vi "Exercise 3-6.vi"() -> ()   [LabVIEW 2014]
panel:
  out "Temperature in Desired Measurement":dbl
  in  "Temperature":dbl
  in  "Desired Measurement":enum16{"K", "F", "C"}(ring)
  in  "Temperature Measurment":enum16{"F", "C"}(ring)
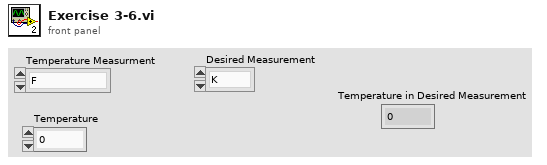
[diagram p1: front panel]
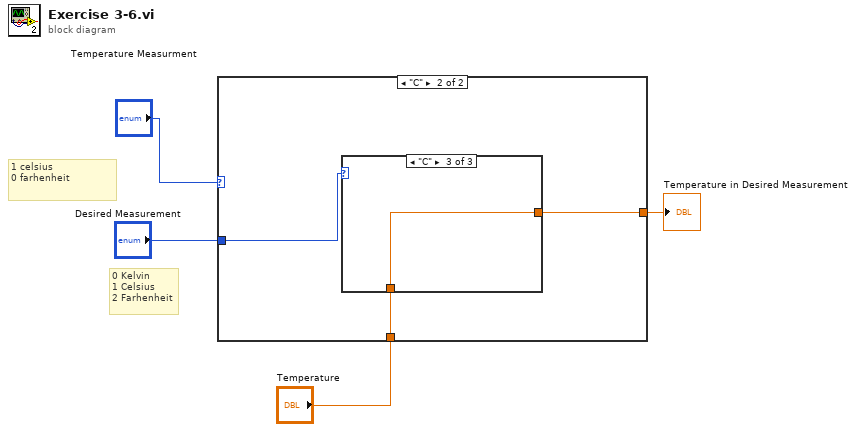
[diagram p0: block diagram]
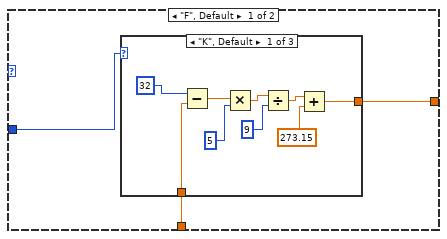
[diagram p2: hidden frame]
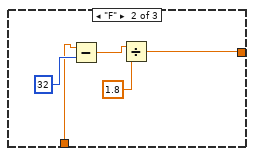
[diagram p3: hidden frame]
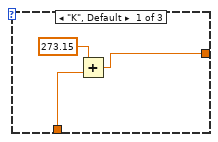
[diagram p5: hidden frame]
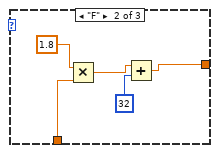
[diagram p6: hidden frame]
diagram:
  # "0 Kelvin\n1 Celsius\n2 Farhenheit"
  # "1 celsius\n0 farhenheit"
  n1 = case shown="\"C\"" "Temperature Measurment" {
    tunnel: "Desired Measurement" -> [w7 w23]
    tunnel: "Temperature" -> [w6 w25]
    tunnel: [w5 w24] -> w2
    frame "F", Default {
      n2 = case shown="\"K\", Default" w7 {
        tunnel: w6 -> [w15 w20 w22]
        tunnel: [w8 w17 w22] -> w5
        frame "K", Default {
          n3 = Subtract(x=32, y=w15) -> (x-y=w14:dbl)
          n4 = Multiply(x=w14, y=5) -> (x*y=w12:dbl)
          n5 = Divide(x=w12, y=9) -> (x/y=w10:dbl)
          n6 = Add(x=w10, y=273.15) -> (x+y=w8:dbl)
        }
        frame "F" {
          n7 = Subtract(x=w20, y=32) -> (x-y=w19:dbl)
          n8 = Divide(x=w19, y=1.8) -> (x/y=w17:dbl)
        }
        frame "C" {
        }
      }
    }
    frame "C" {
      n9 = case shown="\"C\"" w23 {
        tunnel: w25 -> [w27 w32 w34]
        tunnel: [w26 w29 w34] -> w24
        frame "K", Default {
          n10 = Add(x=273.15, y=w27) -> (x+y=w26:dbl)
        }
        frame "F" {
          n11 = Multiply(x=1.8, y=w32) -> (x*y=w30:dbl)
          n12 = Add(x=w30, y=32) -> (x+y=w29:dbl)
        }
        frame "C" {
        }
      }
    }
  }
  "Temperature in Desired Measurement" <- w2
